vi "Configure UL-DL Periodicity.vi"(8 "error in (no error)":errorcluster, 9 "Periodicity (2 ms)":i32(ring)=4 items=["0.5 ms", "0.625 ms", "1 ms", "1.25 ms", "2 ms", "2.5 ms", "5 ms", "10 ms"], 10 "Instance (1)":T1=1, 11 "VISA resource name":refnum<visa-resource-name>) -> (0 "error out":errorcluster, 3 "VISA resource name out":refnum<visa-resource-name>)   [LabVIEW 2020, in "Rohde&Schwarz CMXP NR FR2 Measurement.lvlib"]
doc: "Configures the periodicity of the UL-DL pattern.\n\nAttribute:\nRSCMXPNRFR2M_ATTR_UL_DL_PERIODICITY\n\nRemote-control command:\nCONFigure:NRMMw:MEAS<i>:ULDL:PERiodicity"
uses:
  <instrlib>/Rohde&Schwarz CMXP NR FR2 Measurement/Rohde&Schwarz CMXP NR FR2 Measurement.lvlib
  <instrlib>/Rohde&Schwarz CMXP NR FR2 Measurement/Private/_Instance.ctl
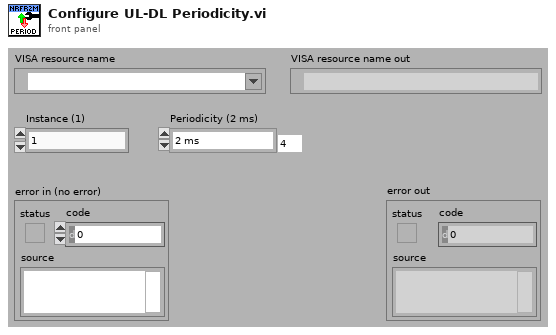
[diagram p1: front panel]
types:
  T1 = typedef "Rohde&Schwarz CMXP NR FR2 Measurement.lvlib/_Instance.ctl" = i32
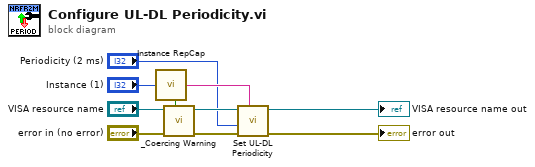
[diagram p0: block diagram]
diagram:
  n1 = call <instrlib>:"Instance RepCap.vi"("Instance In"="Instance (1)") -> ("In Range?"=w6:bool, "RepCap Identifier Out"=w3:string)  [unwired: 1 in]
  n2 = call <instrlib>:"_Coercing Warning.vi"("In Range?"=w6, "error in (no error)"="error in (no error)", "VISA resource name"="VISA resource name") -> ("error out"=w4:errorcluster, "VISA resource name out"=w5:refnum<visa-resource-name>)  [unwired: 7 in]
  n3 = call "Set UL-DL Periodicity"("Repeated Capabilities"=w3, "error in (no error)"=w4, "UL-DL Periodicity (0 - 0.5 ms)"="Periodicity (2 ms)", "instrument handle"=w5) -> ("error out"=→"error out":errorcluster, "instrument handle out"=→"VISA resource name out":refnum<visa-resource-name>)  [unwired: 6 in]
